vi "Manual_Control.vi"() -> ()   [LabVIEW 2013]
uses:
  <vilib>/LabVIEW Interface for Arduino/Type Defs/Pin Mode.ctl
  <vilib>/LabVIEW Interface for Arduino/LabVIEW Interface for Arduino.lvlib
panel:
  in  "Sentido 3":bool
  in  "Sentido 2":bool
  in  "Sentido 1":bool
  out "Potenciómetro 1":dbl(knob) scale=0.0..5.0
  out "Potenciómetro 2":dbl(knob) scale=0.0..5.0
  out "Potenciómetro 3":dbl(knob) scale=0.0..5.0
  in  "Velocidad MOTOR 3":u8(knob) scale=0.0..255.0
  in  "Velocidad MOTOR 2":u8(knob) scale=0.0..255.0
  in  "Velocidad MOTOR 1":u8(knob) scale=0.0..255.0
  out "Pinza":dbl(knob) scale=0.0..100.0
  in  "Ángulo Pinza":dbl(knob) scale=0.0..100.0
  in  "STOP":bool
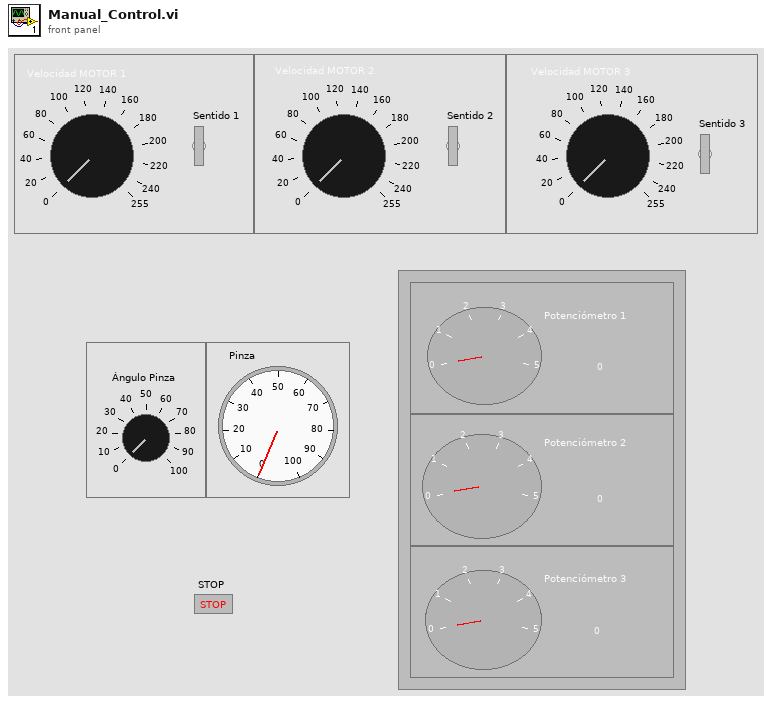
[diagram p1: front panel]
types:
  T1 = typedef "LabVIEW Interface for Arduino.lvlib/Pin Mode.ctl" = enum8{"Input", "Output"}
  T2 = typedef "LabVIEW Interface for Arduino.lvlib/Arduino Resource.ctl" = cluster{"VISA resource":refnum<visa-resource-name>, "Board Type":T3, "Connection Type":enum8{"USB / Serial"}, "Bytes Per Packet (15)":u8}
  T3 = typedef "LabVIEW Interface for Arduino.lvlib/Board Type.ctl" = enum16{"Uno", "Dimuelanove w/Atmega 328", "Mega 2560"}
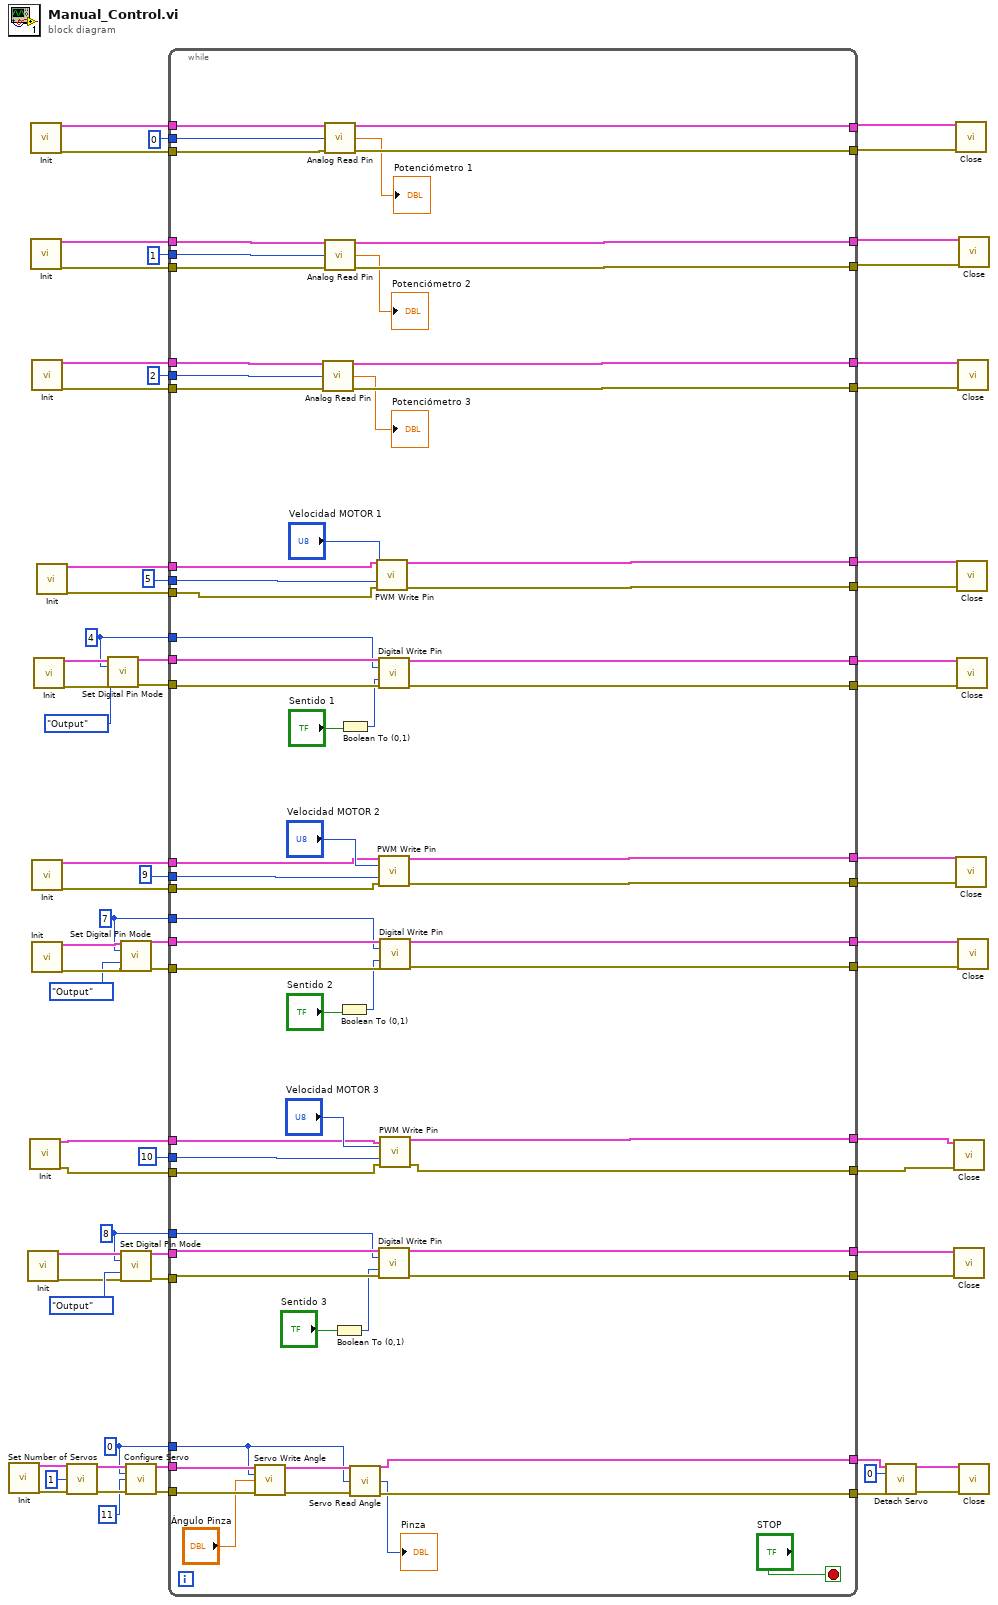
[diagram p0: block diagram]
diagram:
  w3 = u8 8 ("Digital I/O Pin")
  w11 = u8 7 ("Digital I/O Pin")
  w19 = u8 4 ("Digital I/O Pin")
  w60 = u8 0 ("Servo Number (0)")
  n1 = call <vilib>:"Init.vi"() -> ("Arduino Resource"=w68:T2, "error out"=w67:errorcluster)  [unwired: 18 in]
  n2 = call <vilib>:"Init.vi"() -> ("Arduino Resource"=w8:T2, "error out"=w6:errorcluster)  [unwired: 18 in]
  n3 = call <vilib>:"Init.vi"() -> ("Arduino Resource"=w46:T2, "error out"=w45:errorcluster)  [unwired: 18 in]
  n4 = call <vilib>:"Init.vi"() -> ("Arduino Resource"=w29:T2, "error out"=w28:errorcluster)  [unwired: 18 in]
  n5 = call <vilib>:"Init.vi"() -> ("Arduino Resource"=w34:T2, "error out"=w33:errorcluster)  [unwired: 18 in]
  n6 = call <vilib>:"Init.vi"() -> ("Arduino Resource"=w42:T2, "error out"=w41:errorcluster)  [unwired: 18 in]
  n7 = call <vilib>:"Init.vi"() -> ("Arduino Resource"=w50:T2, "error out"=w49:errorcluster)  [unwired: 18 in]
  n8 = call <vilib>:"Init.vi"() -> ("Arduino Resource"=w16:T2, "error out"=w15:errorcluster)  [unwired: 18 in]
  n9 = call <vilib>:"Init.vi"() -> ("Arduino Resource"=w23:T2, "error out"=w22:errorcluster)  [unwired: 18 in]
  n10 = call <vilib>:"Init.vi"() -> ("Arduino Resource"=w54:T2, "error out"=w53:errorcluster)  [unwired: 18 in]
  n11 = call <vilib>:"Set Number of Servos.vi"("Arduino Resource"=w68, "Number Of Servos (1)"=u8 1, "error in"=w67) -> ("Arduino Resource"=w65:T2, "error out"=w64:errorcluster)  [unwired: 11 in]
  n12 = call <vilib>:"Set Digital Pin Mode.vi"("Arduino Resource"=w23, "Digital I/O Pin"=w19, "Pin Mode (Input)"=Pin_Mode."Output", "error in"=w22) -> ("Arduino Resource"=w21:T2, "error out"=w20:errorcluster)  [unwired: 10 in]
  n13 = call <vilib>:"Set Digital Pin Mode.vi"("Arduino Resource"=w16, "Digital I/O Pin"=w11, "Pin Mode (Input)"=Pin_Mode."Output", "error in"=w15) -> ("Arduino Resource"=w13:T2, "error out"=w12:errorcluster)  [unwired: 10 in]
  n14 = call <vilib>:"Set Digital Pin Mode.vi"("Arduino Resource"=w8, "Digital I/O Pin"=w3, "Pin Mode (Input)"=Pin_Mode."Output", "error in"=w6) -> ("Arduino Resource"=w5:T2, "error out"=w4:errorcluster)  [unwired: 10 in]
  n15 = call <vilib>:"Configure Servo.vi"("Arduino Resource"=w65, "Servo Number (0)"=w60, "DIO Pin (2)"=u8 11, "error in"=w64) -> ("Arduino Resource"=w62:T2, "error out"=w61:errorcluster)  [unwired: 10 in]
  n16 = while {
    tunnel: w62 -> [w134]
    tunnel: w61 -> [w133]
    tunnel: w60 -> [w130]
    tunnel: [w129] -> w58
    tunnel: [w128] -> w57
    tunnel: w54 -> [w125]
    tunnel: w53 -> [w124]
    tunnel: [w122] -> w52
    tunnel: [w121] -> w51
    tunnel: w50 -> [w119]
    tunnel: w49 -> [w118]
    tunnel: [w117] -> w48
    tunnel: [w116] -> w47
    tunnel: w46 -> [w114]
    tunnel: w45 -> [w113]
    tunnel: [w112] -> w44
    tunnel: [w111] -> w43
    tunnel: w42 -> [w107]
    tunnel: w41 -> [w106]
    tunnel: u8 5 ("PWM Pin (3)") -> [w110]
    tunnel: u8 9 ("PWM Pin (3)") -> [w109]
    tunnel: u8 10 ("PWM Pin (3)") -> [w108]
    tunnel: u8 2 ("Analog Input Pin (0)") -> [w105]
    tunnel: [w104] -> w36
    tunnel: [w103] -> w35
    tunnel: w34 -> [w101]
    tunnel: w33 -> [w100]
    tunnel: u8 1 ("Analog Input Pin (0)") -> [w99]
    tunnel: [w98] -> w31
    tunnel: [w97] -> w30
    tunnel: w29 -> [w95]
    tunnel: w28 -> [w94]
    tunnel: [w93] -> w26
    tunnel: [w92] -> w25
    tunnel: u8 0 ("Analog Input Pin (0)") -> [w91]
    tunnel: w21 -> [w89]
    tunnel: w20 -> [w88]
    tunnel: w19 -> [w87]
    tunnel: [w84] -> w18
    tunnel: [w83] -> w17
    tunnel: w13 -> [w82]
    tunnel: w12 -> [w81]
    tunnel: w11 -> [w80]
    tunnel: [w77] -> w10
    tunnel: [w76] -> w9
    tunnel: w5 -> [w75]
    tunnel: w4 -> [w74]
    tunnel: w3 -> [w73]
    tunnel: [w70] -> w2
    tunnel: [w69] -> w1
    stop <- "STOP" stop-if-true
    n17 = call <vilib>:"Servo Write Angle.vi"("Arduino Resource"=w134, "Servo Number"=w130, "Angle (Degrees)"="Ángulo Pinza", "error in"=w133) -> ("Arduino Resource"=w132:T2, "error out"=w131:errorcluster)  [unwired: 10 in]
    n18 = call <vilib>:"Analog Read Pin.vi"("Arduino Resource"=w107, "Analog Input Pin (0)"=w105, "error in"=w106) -> ("Arduino Resource"=w104:T2, "Voltage"=→"Potenciómetro 3":dbl, "error out"=w103:errorcluster)  [unwired: 10 in]
    n19 = call <vilib>:"Analog Read Pin.vi"("Arduino Resource"=w95, "Analog Input Pin (0)"=w91, "error in"=w94) -> ("Arduino Resource"=w93:T2, "Voltage"=→"Potenciómetro 1":dbl, "error out"=w92:errorcluster)  [unwired: 10 in]
    n20 = call <vilib>:"Analog Read Pin.vi"("Arduino Resource"=w101, "Analog Input Pin (0)"=w99, "error in"=w100) -> ("Arduino Resource"=w98:T2, "Voltage"=→"Potenciómetro 2":dbl, "error out"=w97:errorcluster)  [unwired: 10 in]
    n21 = Boolean To (0,1)(Boolean="Sentido 3") -> (0, 1=w71:i16)
    n22 = Boolean To (0,1)(Boolean="Sentido 2") -> (0, 1=w78:i16)
    n23 = Boolean To (0,1)(Boolean="Sentido 1") -> (0, 1=w85:i16)
    n24 = call <vilib>:"Servo Read Angle.vi"("Arduino Resource"=w132, "Servo Number"=w130, "error in"=w131) -> ("Arduino Resource"=w129:T2, "Angle (Degrees)"=→"Pinza":u8, "error out"=w128:errorcluster)  [unwired: 10 in]
    n25 = call <vilib>:"PWM Write Pin.vi"("Arduino Resource"=w125, "Duty Cycle (0 - 255)"="Velocidad MOTOR 1", "PWM Pin (3)"=w110, "error in"=w124) -> ("Arduino Resource"=w122:T2, "error out"=w121:errorcluster)  [unwired: 10 in]
    n26 = call <vilib>:"Digital Write Pin.vi"("Arduino Resource"=w89, "Digital I/O Pin (0)"=w87, "Value (0)"=w85, "error in"=w88) -> ("Arduino Resource"=w84:T2, "error out"=w83:errorcluster)  [unwired: 10 in]
    n27 = call <vilib>:"PWM Write Pin.vi"("Arduino Resource"=w119, "Duty Cycle (0 - 255)"="Velocidad MOTOR 2", "PWM Pin (3)"=w109, "error in"=w118) -> ("Arduino Resource"=w117:T2, "error out"=w116:errorcluster)  [unwired: 10 in]
    n28 = call <vilib>:"Digital Write Pin.vi"("Arduino Resource"=w75, "Digital I/O Pin (0)"=w73, "Value (0)"=w71, "error in"=w74) -> ("Arduino Resource"=w70:T2, "error out"=w69:errorcluster)  [unwired: 10 in]
    n29 = call <vilib>:"Digital Write Pin.vi"("Arduino Resource"=w82, "Digital I/O Pin (0)"=w80, "Value (0)"=w78, "error in"=w81) -> ("Arduino Resource"=w77:T2, "error out"=w76:errorcluster)  [unwired: 10 in]
    n30 = call <vilib>:"PWM Write Pin.vi"("Arduino Resource"=w114, "Duty Cycle (0 - 255)"="Velocidad MOTOR 3", "PWM Pin (3)"=w108, "error in"=w113) -> ("Arduino Resource"=w112:T2, "error out"=w111:errorcluster)  [unwired: 10 in]
  }
  n31 = call <vilib>:"Detach Servo.vi"("Arduino Resource"=w58, "Servo Number"=u8 0, "error in"=w57) -> ("Arduino Resource"=w56:T2, "error out"=w55:errorcluster)  [unwired: 11 in]
  n32 = call <vilib>:"Close.vi"("Arduino Resource"=w44, "error in"=w43) -> ()  [unwired: 13 in, 1 out]
  n33 = call <vilib>:"Close.vi"("Arduino Resource"=w2, "error in"=w1) -> ()  [unwired: 13 in, 1 out]
  n34 = call <vilib>:"Close.vi"("Arduino Resource"=w26, "error in"=w25) -> ()  [unwired: 13 in, 1 out]
  n35 = call <vilib>:"Close.vi"("Arduino Resource"=w48, "error in"=w47) -> ()  [unwired: 13 in, 1 out]
  n36 = call <vilib>:"Close.vi"("Arduino Resource"=w52, "error in"=w51) -> ()  [unwired: 13 in, 1 out]
  n37 = call <vilib>:"Close.vi"("Arduino Resource"=w18, "error in"=w17) -> ()  [unwired: 13 in, 1 out]
  n38 = call <vilib>:"Close.vi"("Arduino Resource"=w36, "error in"=w35) -> ()  [unwired: 13 in, 1 out]
  n39 = call <vilib>:"Close.vi"("Arduino Resource"=w10, "error in"=w9) -> ()  [unwired: 13 in, 1 out]
  n40 = call <vilib>:"Close.vi"("Arduino Resource"=w31, "error in"=w30) -> ()  [unwired: 13 in, 1 out]
  n41 = call <vilib>:"Close.vi"("Arduino Resource"=w56, "error in"=w55) -> ()  [unwired: 13 in, 1 out]
